vi "ParseCSV.vi"(8 "error in (no error)":errorcluster, 11 "Target Path":path) -> (0 "error out":errorcluster, 3 "Zone Setup Array":cluster{"Zone Selector":string, "Timing":dbl}[](array[cluster]))   [LabVIEW 2019]
uses:
  <vilib>/Utility/file.llb/Read Delimited Spreadsheet (string).vi
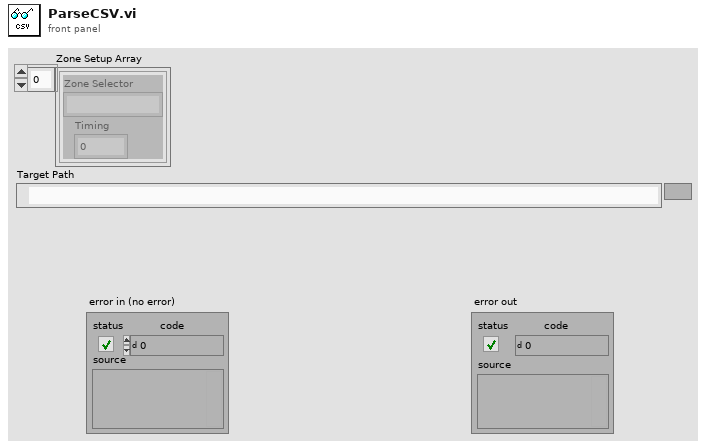
[diagram p1: front panel]
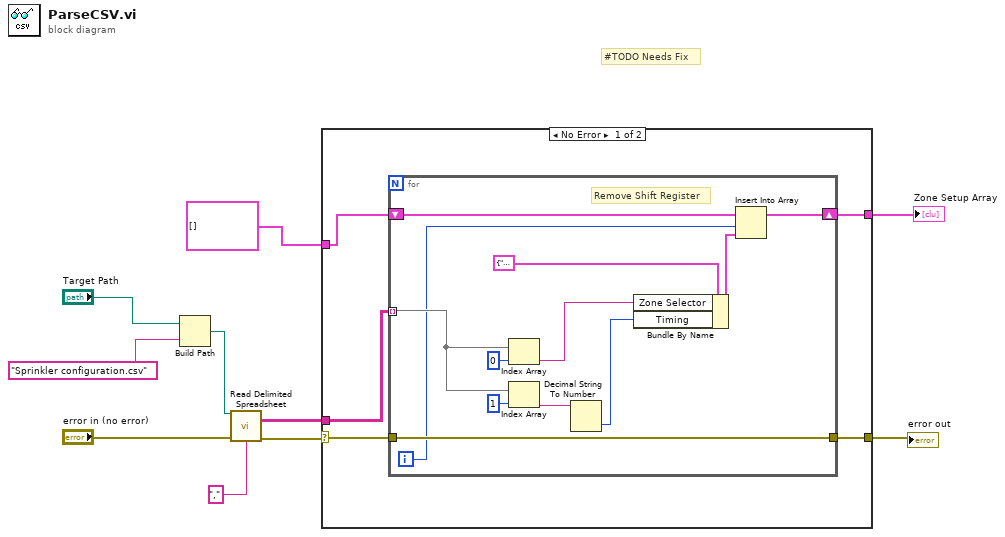
[diagram p0: block diagram]
diagram:
  # "#TODO Needs Fix"
  n1 = Build Path(base path="Target Path", name or relative path="Sprinkler configuration.csv") -> (appended path=w7:path)
  n2 = call-poly <vilib>:"Read Delimited Spreadsheet.vi"("file path (dialog if empty)"=w7, "error in (no error)"="error in (no error)", "delimiter (\\t)"="," ("delimiter (\\t)")) -> ("all rows"=w6:string[][], "error out"=w8:errorcluster)  [unwired: 7 in, 4 out]
  n3 = case shown="No Error" w8 {
    selector: w8 -> [w14 w28]
    tunnel: w6 -> [w15 _]
    tunnel: cluster{"Zone Selector":string, "Timing":dbl}[] [] ("Zone Setup Array") -> [w13 w29]
    tunnel: [w11 w29] -> w4
    tunnel: [w12 w28] -> w3
    frame No Error {
      n4 = for {
        tunnel: w15 -> [w26] mode=indexing
        tunnel: w14 -> [w27]
        tunnel: [w27] -> w12
        shift-right: [w16] -> w11
        shift-left: w13 -> [w23]
        i -> [w22]
        # "Remove Shift Register"
        n5 = Index Array(array=w26, index=0) -> (element=w19:string)
        n6 = Index Array(array=w26, index=1) -> (element=w20:string)
        n7 = Decimal String To Number(string=w20) -> (number=w18:i32)  [unwired: 2 in, 1 out]
        n8 = Bundle By Name(cluster=cluster{"Zone Selector":string, "Timing":dbl} {"Zone Selector"="", "Timing"=0.0} ("Zone Selector"), "Zone Selector"=w19, "Timing"=w18) -> (w17:cluster{"Zone Selector":string, "Timing":dbl})
        n9 = Insert Into Array "Insert Into Array"(array=w23, index=w22, new element=w17) -> (w16:cluster{"Zone Selector":string, "Timing":dbl}[])
      }
    }
    frame Error {
    }
  }
  "error out" <- w3
  "Zone Setup Array" <- w4
